vi "GSM调试.vi"() -> ()   [LabVIEW 2015]
doc: "GSM调试"
uses:
  <vilib>/Platform/browser.llb/Open URL in Default Browser (string).vi
  lib/pcomm/PCOMM.lvlib
panel:
  out "字符串 4":string="通用指令"
  out "字符串 3":string="串口设置"
  in  "刷新按钮":bool
  out "字符串 2":string="串口设置"
  in  "发送":string
  in  "打开/关闭串口":bool
  in  "波特率":i32(ring)=16 items=["1800"=8, "2400"=9, "4800"=10, "7200"=11, "9600"=12, "19200"=13, "38400"=14, "57600"=15, "115200"=16, "230400"=17, "460800"=18, "921600"=19]
  in  "数据比特":i32(ring)=3 caption="数据位" items=["5", "6", "7", "8"]
  in  "停止位":i32(ring) items=["1"=0, "2"=4]
  in  "奇偶校验":i32(ring) caption="校   验" items=["None"=0, "Odd"=8, "Even"=24, "Mark"=40, "Space"=56]
  in  "串口号":i32(ring)=1 items=["COM1 通信端口 (COM1)"=1, "COM2 ELTIMA Virtual Serial Port (COM2->COM5)"=2, "COM4 USB-SERIAL CH340 (COM4)"=4, "COM5 ELTIMA Virtual Serial Port (COM5->COM2)"=5]
  in  "打开文档":bool
  in  "清屏":bool
  in  "编号":u16
  in  "短信":string
  in  "号码":u64
  in  "显示回车换行":bool
  in  "GSM指令":T1={"响应测试"=FALSE, "版本信息"=FALSE, "查询IMEI"=FALSE, "信号质量查询"=FALSE, "本机号码"=FALSE, "显示ID"=FALSE, "呼叫号码"=FALSE, "查询短信状态"=FALSE, "查询温度"=FALSE, "查询音量"=FALSE, "默认配置"=FALSE, "查询运营商"=FALSE, "当前配置"=FALSE, "查询型号"=FALSE, "接听电话"=FALSE, "挂断电话"=FALSE, "读取短信"=FALSE, "删除短信"=FALSE, "删除全部短信"=FALSE, "发送短信"=FALSE, "信息显示"="", "字符串 4"="通用指令", "字符串 5"="通用指令"}
  out "接收文本框:":string
  out "TX:":i32 max=65535
  out "RX:":i32 max=1000
  in  "发送":bool
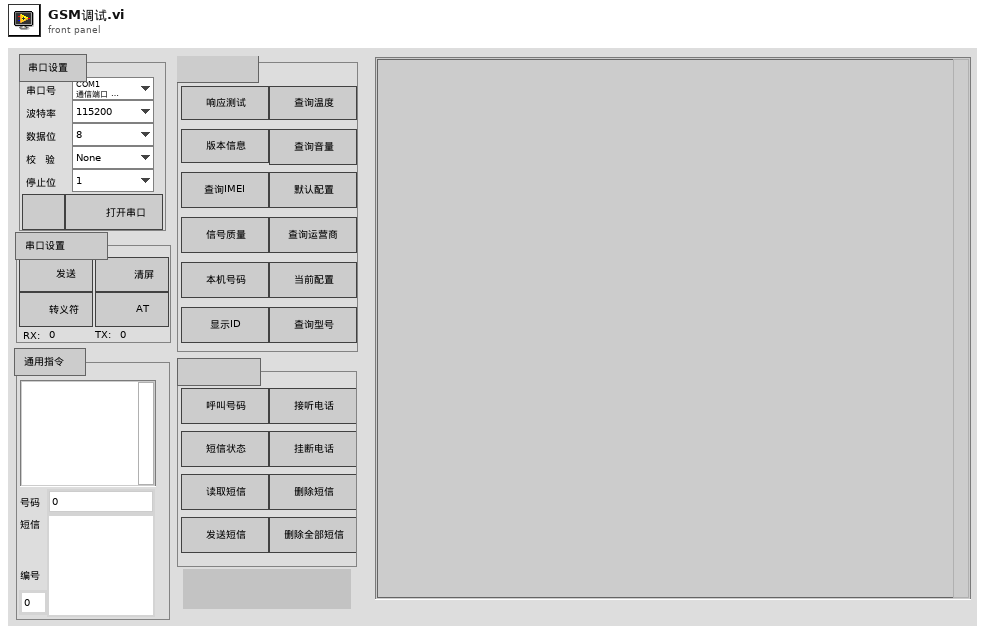
[diagram p1: front panel]
types:
  T1 = cluster{"响应测试":bool, "版本信息":bool, "查询IMEI":bool, "信号质量查询":bool, "本机号码":bool, "显示ID":bool, "呼叫号码":bool, "查询短信状态":bool, "查询温度":bool, "查询音量":bool, "默认配置":bool, "查询运营商":bool, "当前配置":bool, "查询型号":bool, "接听电话":bool, "挂断电话":bool, "读取短信":bool, "删除短信":bool, "删除全部短信":bool, "发送短信":bool, "信息显示":string, "字符串 4":string, "字符串 5":string}
  T2 = enum8{"Enabled", "Disabled", "Disabled and Grayed Out"}
  T3 = typedef "LVRectTypeDef.ctl" = cluster{"Left":i16, "Top":i16, "Right":i16, "Bottom":i16}
  T4 = typedef "LVPointTypeDef.ctl" = cluster{"Horizontal":i16, "Vertical":i16}
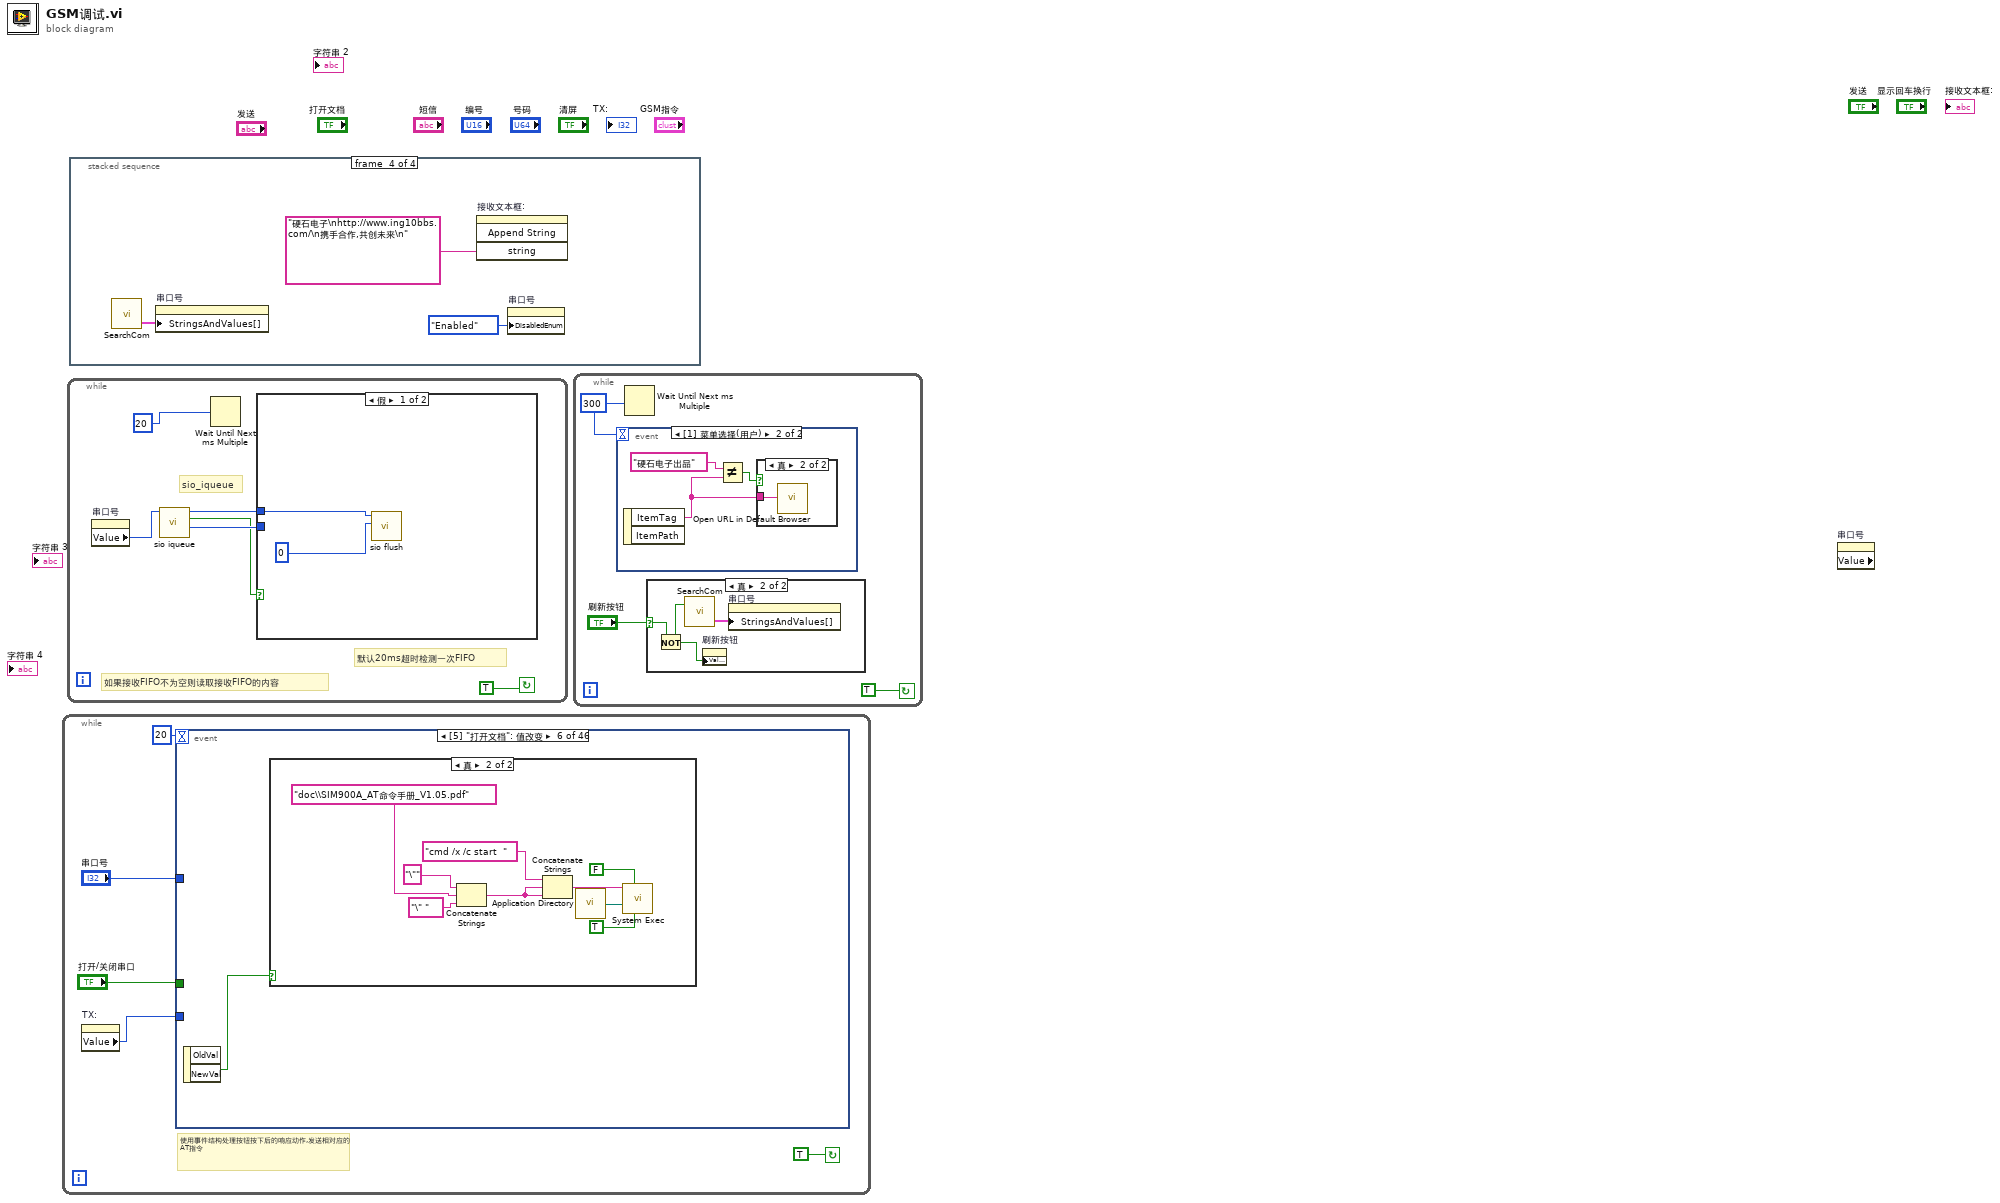
[diagram p0: block diagram]
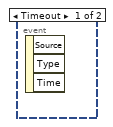
[diagram p3: hidden frame]
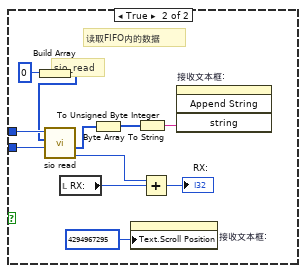
[diagram p5: hidden frame]
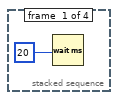
[diagram p6: hidden frame]
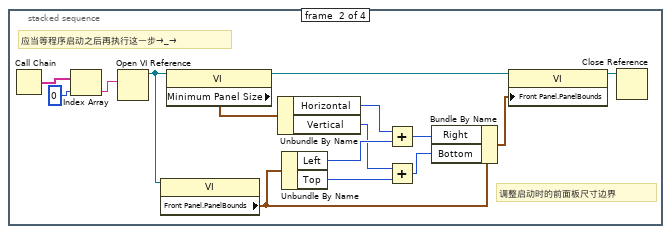
[diagram p7: hidden frame]
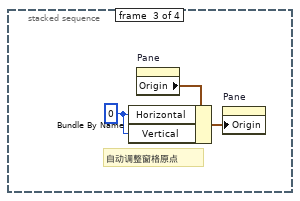
[diagram p8: hidden frame]
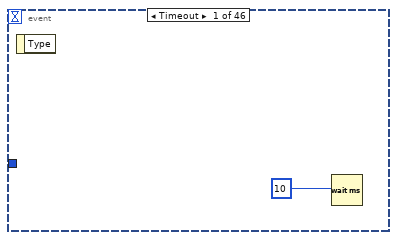
[diagram p9: hidden frame]
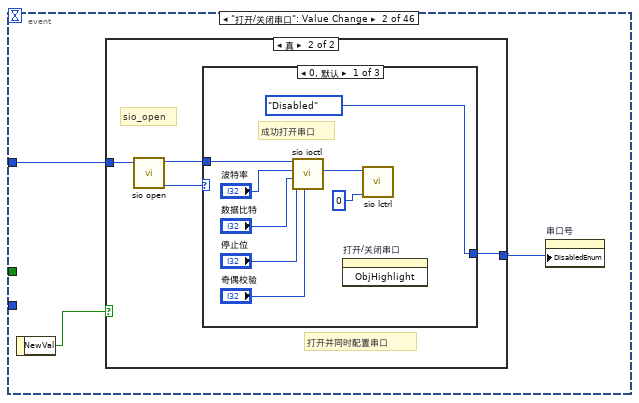
[diagram p10: hidden frame]
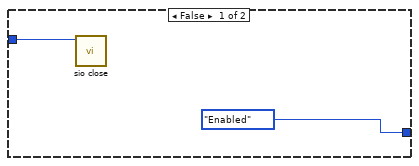
[diagram p11: hidden frame]
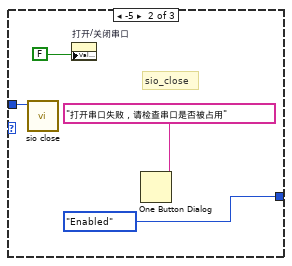
[diagram p12: hidden frame]
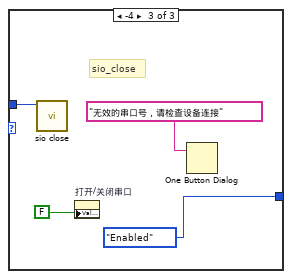
[diagram p13: hidden frame]
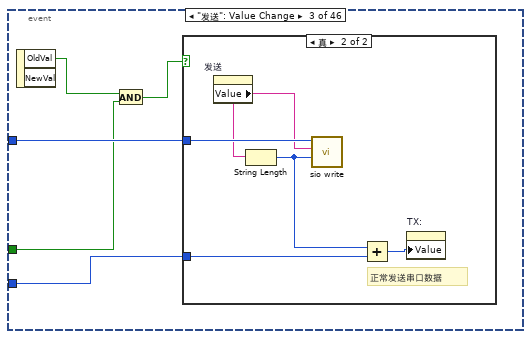
[diagram p14: hidden frame]
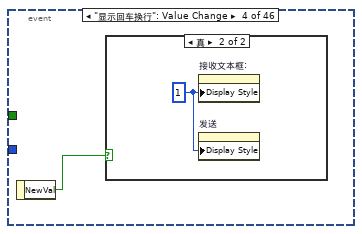
[diagram p16: hidden frame]
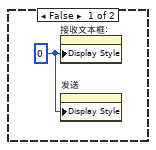
[diagram p17: hidden frame]
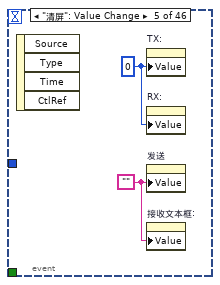
[diagram p18: hidden frame]
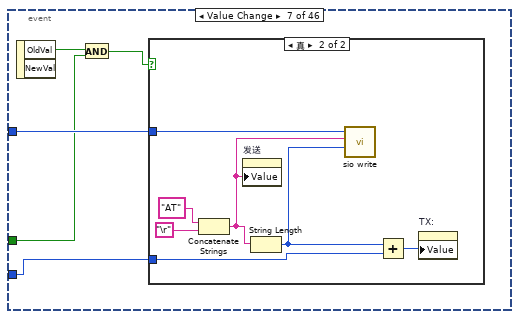
[diagram p20: hidden frame]
diagram:
  n1 = while {
    stop <- TRUE continue-if-true
    # "使用事件结构处理按钮按下后的响应动作,发送相对应的AT指令"
    n2 = property on="TX:" class="DigNum (严格)"() -> ("Value"=w4:i32)  [unwired: 2 in, 2 out]
    n3 = event shown="[5] \"打开文档\": 值改变" {
      selector: _ -> [_ _ _ _ _ _ _ _ _ _ _ _ _ _ _ _ _ _ _ _ _ _ _ _ _ _ _ _ _ _ _ _ _ _ _ _ _ _ _ _ _ _ _ _ _ _]
      dyn-events: _ -> [_ _ _ _ _ _ _ _ _ _ _ _ _ _ _ _ _ _ _ _ _ _ _ _ _ _ _ _ _ _ _ _ _ _ _ _ _ _ _ _ _ _ _ _ _ _]
      timeout: 20 -> [_ _ _ _ _ _ _ _ _ _ _ _ _ _ _ _ _ _ _ _ _ _ _ _ _ _ _ _ _ _ _ _ _ _ _ _ _ _ _ _ _ _ _ _ _ _]
      tunnel: w4 -> [_ _ w36 _ _ _ w61 w73 w85 w97 w109 w121 w133 w148 w160 w172 w184 w196 w208 w220 w232 w244 w256 w270 w284 w295 _ _ _ _ _ _ _ _ _ _ _ _ _ _ _ _ _ _ _ _]
      tunnel: "串口号" -> [_ w8 w35 _ _ _ w60 w72 w84 w96 w108 w120 w132 w147 w159 w171 w183 w195 w207 w219 w231 w243 w255 w269 w283 w296 _ _ _ _ _ _ _ _ _ _ _ _ _ _ _ _ _ _ _ _]
      tunnel: "打开/关闭串口" -> [_ _ w33 _ _ _ w58 w70 w82 w94 w106 w118 w130 w145 w157 w169 w181 w193 w205 w217 w229 w241 w253 w267 w281 w293 _ _ _ _ _ _ _ _ _ _ _ _ _ _ _ _ _ _ _ _]
      event Timeout {
        n4 = event-data() -> ()  [unwired: 1 in, 1 out]
        n5 = Wait (ms)(milliseconds to wait=10) -> ()  [unwired: 1 out]
      }
      event "打开/关闭串口": Value Change {
        n6 = event-data() -> ("NewVal"=w9:bool)  [unwired: 1 in]
        n7 = case shown="真" w9 {
          tunnel: w8 -> [w10 w12]
          tunnel: [T2."Enabled" w13] -> w7
          frame False {
            n8 = call "sio close.vi"("port"=w10) -> ()  [unwired: 9 in, 2 out]
          }
          frame True {
            # "sio_open"
            # "打开并同时配置串口"
            n9 = call "sio open.vi"("port"=w12) -> ("port"=w14:i32, "Status"=w15:i32)  [unwired: 6 in]
            n10 = case shown="0, 默认" w15 {
              tunnel: w14 -> [w19 w24 w28]
              tunnel: [T2."Disabled" T2."Enabled" T2."Enabled"] -> w13
              frame 0, Default {
                # "成功打开串口"
                n11 = call "sio ioctl.vi"("parity"="奇偶校验", "stop bits"="停止位", "data bits"="数据比特", "baud"="波特率", "port"=w19) -> ("port"=w17:i32)  [unwired: 5 in, 1 out]
                n12 = invoke on="打开/关闭串口" class="Bool (严格)" method="ObjHighlight"() -> ()  [unwired: 3 in, 3 out]
                n13 = call "sio lctrl.vi"("mode"=0, "port"=w17) -> ()  [unwired: 8 in, 2 out]
              }
              frame -5 {
                # "sio_close"
                n14 = call "sio close.vi"("port"=w24) -> ()  [unwired: 9 in, 2 out]
                n15 = property on="打开/关闭串口" class="Bool (严格)"("Value"=FALSE) -> ()  [unwired: 2 in, 2 out]
                n16 = One Button Dialog(message="打开串口失败，请检查串口是否被占用") -> ()  [unwired: 1 in, 1 out]
              }
              frame -4 {
                # "sio_close"
                n17 = call "sio close.vi"("port"=w28) -> ()  [unwired: 9 in, 2 out]
                n18 = property on="打开/关闭串口" class="Bool (严格)"("Value"=FALSE) -> ()  [unwired: 2 in, 2 out]
                n19 = One Button Dialog(message="无效的串口号，请检查设备连接") -> ()  [unwired: 1 in, 1 out]
              }
            }
          }
        }
        n20 = property on="串口号" class="Ring (严格)"("DisabledEnum"=w7) -> ()  [unwired: 2 in, 2 out]
      }
      event "发送": Value Change {
        n21 = event-data() -> ("OldVal"=w34:bool)  [unwired: 1 in, 1 out]
        n22 = And(x=w34, y=w33) -> (x .and. y?=w32:bool)
        n23 = case shown="真" w32 {
          tunnel: w35 -> [_ w39]
          tunnel: w36 -> [_ w41]
          frame False {
          }
          frame True {
            # "正常发送串口数据"
            n24 = property on="发送" class="Str"() -> ("Value"=w38:string)  [unwired: 2 in, 2 out]
            n25 = String Length(string=w38) -> (length=w37:i32)
            n26 = call "sio write.vi"("len"=w37, "buf"=w38, "port"=w39) -> ()  [unwired: 6 in, 3 out]
            n27 = Add(x=w37, y=w41) -> (x+y=w40:i32)
            n28 = property on="TX:" class="DigNum (严格)"("Value"=w40) -> ()  [unwired: 2 in, 2 out]
          }
        }
      }
      event "显示回车换行": Value Change {
        n29 = event-data() -> ("NewVal"=w42:bool)  [unwired: 1 in]
        n30 = case shown="真" w42 {
          frame False {
            w43 = u32 0
            n31 = property on="接收文本框:" class="Str"("Display Style"=w43) -> ()  [unwired: 2 in, 2 out]
            n32 = property on="发送" class="Str"("Display Style"=w43) -> ()  [unwired: 2 in, 2 out]
          }
          frame True {
            w44 = u32 1
            n33 = property on="接收文本框:" class="Str"("Display Style"=w44) -> ()  [unwired: 2 in, 2 out]
            n34 = property on="发送" class="Str"("Display Style"=w44) -> ()  [unwired: 2 in, 2 out]
          }
        }
      }
      event "清屏": Value Change {
        w45 = ""
        w46 = 0
        n35 = event-data() -> ()  [unwired: 1 in, 4 out]
        n36 = property on="TX:" class="DigNum (严格)"("Value"=w46) -> ()  [unwired: 2 in, 2 out]
        n37 = property on="RX:" class="DigNum (严格)"("Value"=w46) -> ()  [unwired: 2 in, 2 out]
        n38 = property on="发送" class="Str"("Value"=w45) -> ()  [unwired: 2 in, 2 out]
        n39 = property on="接收文本框:" class="Str"("Value"=w45) -> ()  [unwired: 2 in, 2 out]
      }
      event "打开文档": Value Change {
        n40 = event-data() -> ("NewVal"=w47:bool)  [unwired: 1 in, 1 out]
        n41 = case shown="真" w47 {
          frame False {
          }
          frame True {
            n42 = Concatenate Strings("\"" ("Substring"), "doc\\SIM900A_AT命令手册_V1.05.pdf", "\" " ("Substring")) -> (w53:string)
            n43 = Concatenate Strings("cmd /x /c start  ", w53, w53) -> (w55:string)
            n44 = call <vilib>:"Application Directory.vi"() -> ("Application Directory"=w48:path)
            n45 = call <vilib>:"System Exec.vi"("run minimized? (F)"=TRUE, "wait until completion? (T)"=FALSE ("Wait until done"), "working directory"=w48, "command line"=w55) -> ()  [unwired: 2 in, 6 out]
          }
        }
      }
      event "GSM指令.响应测试": Value Change {
        n46 = event-data() -> ("OldVal"=w59:bool)  [unwired: 1 in, 1 out]
        n47 = And(x=w59, y=w58) -> (x .and. y?=w57:bool)
        n48 = case shown="真" w57 {
          tunnel: w60 -> [_ w64]
          tunnel: w61 -> [_ w67]
          frame False {
          }
          frame True {
            n49 = Concatenate Strings("AT", "\r") -> (w63:string)
            n50 = property on="发送" class="Str"("Value"=w63) -> ()  [unwired: 2 in, 2 out]
            n51 = String Length(string=w63) -> (length=w62:i32)
            n52 = call "sio write.vi"("len"=w62, "buf"=w63, "port"=w64) -> ()  [unwired: 6 in, 3 out]
            n53 = Add(x=w62, y=w67) -> (x+y=w68:i32)
            n54 = property on="TX:" class="DigNum (严格)"("Value"=w68) -> ()  [unwired: 2 in, 2 out]
          }
        }
      }
      event "GSM指令.版本信息": Value Change {
        n55 = event-data() -> ("OldVal"=w69:bool)  [unwired: 1 in, 1 out]
        n56 = And(x=w70, y=w69) -> (x .and. y?=w71:bool)
        n57 = case shown="真" w71 {
          tunnel: w72 -> [_ w76]
          tunnel: w73 -> [_ w79]
          frame False {
          }
          frame True {
            n58 = Concatenate Strings("AT+GSV", "\r") -> (w75:string)
            n59 = property on="发送" class="Str"("Value"=w75) -> ()  [unwired: 2 in, 2 out]
            n60 = String Length(string=w75) -> (length=w74:i32)
            n61 = call "sio write.vi"("len"=w74, "buf"=w75, "port"=w76) -> ()  [unwired: 6 in, 3 out]
            n62 = Add(x=w74, y=w79) -> (x+y=w80:i32)
            n63 = property on="TX:" class="DigNum (严格)"("Value"=w80) -> ()  [unwired: 2 in, 2 out]
          }
        }
      }
      event "GSM指令.查询IMEI": Value Change {
        n64 = event-data() -> ("OldVal"=w83:bool)  [unwired: 1 in, 1 out]
        n65 = And(x=w83, y=w82) -> (x .and. y?=w81:bool)
        n66 = case shown="真" w81 {
          tunnel: w84 -> [_ w88]
          tunnel: w85 -> [_ w91]
          frame False {
          }
          frame True {
            n67 = Concatenate Strings("AT+GSN", "\r") -> (w87:string)
            n68 = property on="发送" class="Str"("Value"=w87) -> ()  [unwired: 2 in, 2 out]
            n69 = String Length(string=w87) -> (length=w86:i32)
            n70 = call "sio write.vi"("len"=w86, "buf"=w87, "port"=w88) -> ()  [unwired: 6 in, 3 out]
            n71 = Add(x=w86, y=w91) -> (x+y=w92:i32)
            n72 = property on="TX:" class="DigNum (严格)"("Value"=w92) -> ()  [unwired: 2 in, 2 out]
          }
        }
      }
      event "GSM指令.信号质量查询": Value Change {
        n73 = event-data() -> ("OldVal"=w95:bool)  [unwired: 1 in, 1 out]
        n74 = And(x=w95, y=w94) -> (x .and. y?=w93:bool)
        n75 = case shown="真" w93 {
          tunnel: w96 -> [_ w100]
          tunnel: w97 -> [_ w103]
          frame False {
          }
          frame True {
            n76 = Concatenate Strings("AT+CSQ", "\r") -> (w99:string)
            n77 = property on="发送" class="Str"("Value"=w99) -> ()  [unwired: 2 in, 2 out]
            n78 = String Length(string=w99) -> (length=w98:i32)
            n79 = call "sio write.vi"("len"=w98, "buf"=w99, "port"=w100) -> ()  [unwired: 6 in, 3 out]
            n80 = Add(x=w98, y=w103) -> (x+y=w104:i32)
            n81 = property on="TX:" class="DigNum (严格)"("Value"=w104) -> ()  [unwired: 2 in, 2 out]
          }
        }
      }
      event "GSM指令.本机号码": Value Change {
        n82 = event-data() -> ("OldVal"=w107:bool)  [unwired: 1 in, 1 out]
        n83 = And(x=w107, y=w106) -> (x .and. y?=w105:bool)
        n84 = case shown="真" w105 {
          tunnel: w108 -> [_ w112]
          tunnel: w109 -> [_ w115]
          frame False {
          }
          frame True {
            n85 = Concatenate Strings("AT+CNUM", "\r") -> (w111:string)
            n86 = String Length(string=w111) -> (length=w110:i32)
            n87 = property on="发送" class="Str"("Value"=w111) -> ()  [unwired: 2 in, 2 out]
            n88 = call "sio write.vi"("len"=w110, "buf"=w111, "port"=w112) -> ()  [unwired: 6 in, 3 out]
            n89 = Add(x=w110, y=w115) -> (x+y=w116:i32)
            n90 = property on="TX:" class="DigNum (严格)"("Value"=w116) -> ()  [unwired: 2 in, 2 out]
          }
        }
      }
      event "GSM指令.显示ID": Value Change {
        n91 = event-data() -> ("OldVal"=w119:bool)  [unwired: 1 in, 1 out]
        n92 = And(x=w119, y=w118) -> (x .and. y?=w117:bool)
        n93 = case shown="真" w117 {
          tunnel: w120 -> [_ w124]
          tunnel: w121 -> [_ w127]
          frame False {
          }
          frame True {
            n94 = Concatenate Strings("ATI", "\r") -> (w123:string)
            n95 = property on="发送" class="Str"("Value"=w123) -> ()  [unwired: 2 in, 2 out]
            n96 = String Length(string=w123) -> (length=w122:i32)
            n97 = call "sio write.vi"("len"=w122, "buf"=w123, "port"=w124) -> ()  [unwired: 6 in, 3 out]
            n98 = Add(x=w122, y=w127) -> (x+y=w128:i32)
            n99 = property on="TX:" class="DigNum (严格)"("Value"=w128) -> ()  [unwired: 2 in, 2 out]
          }
        }
      }
      event "GSM指令.呼叫号码": Value Change {
        n100 = event-data() -> ("OldVal"=w131:bool)  [unwired: 1 in, 1 out]
        n101 = And(x=w131, y=w130) -> (x .and. y?=w129:bool)
        n102 = case shown="真" w129 {
          tunnel: w132 -> [_ w136]
          tunnel: w133 -> [_ w142]
          frame False {
          }
          frame True {
            n103 = property on="号码" class="DigNum (严格)"() -> ("Value"=w138:u64)  [unwired: 2 in, 2 out]
            n104 = Number To Decimal String ("数值至十进制数字符串转换")(number=w138) -> (decimal integer string=w140:string)  [unwired: 1 in]
            n105 = Concatenate Strings("ATD", w140, ";", "\r") -> (w135:string)
            n106 = property on="发送" class="Str"("Value"=w135) -> ()  [unwired: 2 in, 2 out]
            n107 = String Length(string=w135) -> (length=w134:i32)
            n108 = call "sio write.vi"("len"=w134, "buf"=w135, "port"=w136) -> ()  [unwired: 6 in, 3 out]
            n109 = Add(x=w134, y=w142) -> (x+y=w143:i32)
            n110 = property on="TX:" class="DigNum (严格)"("Value"=w143) -> ()  [unwired: 2 in, 2 out]
          }
        }
      }
      event "GSM指令.查询短信状态": Value Change {
        n111 = event-data() -> ("OldVal"=w146:bool)  [unwired: 1 in, 1 out]
        n112 = And(x=w146, y=w145) -> (x .and. y?=w144:bool)
        n113 = case shown="真" w144 {
          tunnel: w147 -> [_ w151]
          tunnel: w148 -> [_ w154]
          frame False {
          }
          frame True {
            n114 = Concatenate Strings("AT+CPMS?", "\r") -> (w150:string)
            n115 = property on="发送" class="Str"("Value"=w150) -> ()  [unwired: 2 in, 2 out]
            n116 = String Length(string=w150) -> (length=w149:i32)
            n117 = Add(x=w149, y=w154) -> (x+y=w155:i32)
            n118 = call "sio write.vi"("len"=w149, "buf"=w150, "port"=w151) -> ()  [unwired: 6 in, 3 out]
            n119 = property on="TX:" class="DigNum (严格)"("Value"=w155) -> ()  [unwired: 2 in, 2 out]
          }
        }
      }
      event "GSM指令.查询温度": Value Change {
        n120 = event-data() -> ("OldVal"=w158:bool)  [unwired: 1 in, 1 out]
        n121 = And(x=w158, y=w157) -> (x .and. y?=w156:bool)
        n122 = case shown="真" w156 {
          tunnel: w159 -> [_ w163]
          tunnel: w160 -> [_ w166]
          frame False {
          }
          frame True {
            n123 = Concatenate Strings("AT+CMTE?", "\r") -> (w162:string)
            n124 = property on="发送" class="Str"("Value"=w162) -> ()  [unwired: 2 in, 2 out]
            n125 = String Length(string=w162) -> (length=w161:i32)
            n126 = Add(x=w161, y=w166) -> (x+y=w167:i32)
            n127 = call "sio write.vi"("len"=w161, "buf"=w162, "port"=w163) -> ()  [unwired: 6 in, 3 out]
            n128 = property on="TX:" class="DigNum (严格)"("Value"=w167) -> ()  [unwired: 2 in, 2 out]
          }
        }
      }
      event "GSM指令.查询音量": Value Change {
        n129 = event-data() -> ("OldVal"=w170:bool)  [unwired: 1 in, 1 out]
        n130 = And(x=w170, y=w169) -> (x .and. y?=w168:bool)
        n131 = case shown="真" w168 {
          tunnel: w171 -> [_ w175]
          tunnel: w172 -> [_ w178]
          frame False {
          }
          frame True {
            n132 = Concatenate Strings("AT+SIDET?", "\r") -> (w174:string)
            n133 = property on="发送" class="Str"("Value"=w174) -> ()  [unwired: 2 in, 2 out]
            n134 = String Length(string=w174) -> (length=w173:i32)
            n135 = call "sio write.vi"("len"=w173, "buf"=w174, "port"=w175) -> ()  [unwired: 6 in, 3 out]
            n136 = Add(x=w173, y=w178) -> (x+y=w179:i32)
            n137 = property on="TX:" class="DigNum (严格)"("Value"=w179) -> ()  [unwired: 2 in, 2 out]
          }
        }
      }
      event "GSM指令.默认配置": Value Change {
        n138 = event-data() -> ("OldVal"=w182:bool)  [unwired: 1 in, 1 out]
        n139 = And(x=w182, y=w181) -> (x .and. y?=w180:bool)
        n140 = case shown="真" w180 {
          tunnel: w183 -> [_ w187]
          tunnel: w184 -> [_ w190]
          frame False {
          }
          frame True {
            n141 = Concatenate Strings("AT&F", "\r") -> (w186:string)
            n142 = property on="发送" class="Str"("Value"=w186) -> ()  [unwired: 2 in, 2 out]
            n143 = String Length(string=w186) -> (length=w185:i32)
            n144 = call "sio write.vi"("len"=w185, "buf"=w186, "port"=w187) -> ()  [unwired: 6 in, 3 out]
            n145 = Add(x=w185, y=w190) -> (x+y=w191:i32)
            n146 = property on="TX:" class="DigNum (严格)"("Value"=w191) -> ()  [unwired: 2 in, 2 out]
          }
        }
      }
      event "GSM指令.查询运营商": Value Change {
        n147 = event-data() -> ("OldVal"=w194:bool)  [unwired: 1 in, 1 out]
        n148 = And(x=w194, y=w193) -> (x .and. y?=w192:bool)
        n149 = case shown="真" w192 {
          tunnel: w195 -> [_ w199]
          tunnel: w196 -> [_ w202]
          frame False {
          }
          frame True {
            n150 = Concatenate Strings("AT+COPS?", "\r") -> (w198:string)
            n151 = property on="发送" class="Str"("Value"=w198) -> ()  [unwired: 2 in, 2 out]
            n152 = String Length(string=w198) -> (length=w197:i32)
            n153 = call "sio write.vi"("len"=w197, "buf"=w198, "port"=w199) -> ()  [unwired: 6 in, 3 out]
            n154 = Add(x=w197, y=w202) -> (x+y=w203:i32)
            n155 = property on="TX:" class="DigNum (严格)"("Value"=w203) -> ()  [unwired: 2 in, 2 out]
          }
        }
      }
      event "GSM指令.当前配置": Value Change {
        n156 = event-data() -> ("OldVal"=w206:bool)  [unwired: 1 in, 1 out]
        n157 = And(x=w206, y=w205) -> (x .and. y?=w204:bool)
        n158 = case shown="真" w204 {
          tunnel: w207 -> [_ w211]
          tunnel: w208 -> [_ w214]
          frame False {
          }
          frame True {
            n159 = Concatenate Strings("AT&V", "\r") -> (w210:string)
            n160 = property on="发送" class="Str"("Value"=w210) -> ()  [unwired: 2 in, 2 out]
            n161 = String Length(string=w210) -> (length=w209:i32)
            n162 = call "sio write.vi"("len"=w209, "buf"=w210, "port"=w211) -> ()  [unwired: 6 in, 3 out]
            n163 = Add(x=w209, y=w214) -> (x+y=w215:i32)
            n164 = property on="TX:" class="DigNum (严格)"("Value"=w215) -> ()  [unwired: 2 in, 2 out]
          }
        }
      }
      event "GSM指令.查询型号": Value Change {
        n165 = event-data() -> ("OldVal"=w218:bool)  [unwired: 1 in, 1 out]
        n166 = And(x=w218, y=w217) -> (x .and. y?=w216:bool)
        n167 = case shown="真" w216 {
          tunnel: w219 -> [_ w223]
          tunnel: w220 -> [_ w226]
          frame False {
          }
          frame True {
            n168 = Concatenate Strings("AT+CGMM", "\r") -> (w222:string)
            n169 = property on="发送" class="Str"("Value"=w222) -> ()  [unwired: 2 in, 2 out]
            n170 = String Length(string=w222) -> (length=w221:i32)
            n171 = call "sio write.vi"("len"=w221, "buf"=w222, "port"=w223) -> ()  [unwired: 6 in, 3 out]
            n172 = Add(x=w221, y=w226) -> (x+y=w227:i32)
            n173 = property on="TX:" class="DigNum (严格)"("Value"=w227) -> ()  [unwired: 2 in, 2 out]
          }
        }
      }
      event "GSM指令.接听电话": Value Change {
        n174 = event-data() -> ("OldVal"=w230:bool)  [unwired: 1 in, 1 out]
        n175 = And(x=w230, y=w229) -> (x .and. y?=w228:bool)
        n176 = case shown="真" w228 {
          tunnel: w232 -> [_ w238]
          tunnel: w231 -> [_ w235]
          frame False {
          }
          frame True {
            n177 = Concatenate Strings("ATA", "\r") -> (w234:string)
            n178 = property on="发送" class="Str"("Value"=w234) -> ()  [unwired: 2 in, 2 out]
            n179 = String Length(string=w234) -> (length=w233:i32)
            n180 = call "sio write.vi"("len"=w233, "buf"=w234, "port"=w235) -> ()  [unwired: 6 in, 3 out]
            n181 = Add(x=w233, y=w238) -> (x+y=w239:i32)
            n182 = property on="TX:" class="DigNum (严格)"("Value"=w239) -> ()  [unwired: 2 in, 2 out]
          }
        }
      }
      event "GSM指令.挂断电话": Value Change {
        n183 = event-data() -> ("OldVal"=w242:bool)  [unwired: 1 in, 1 out]
        n184 = And(x=w242, y=w241) -> (x .and. y?=w240:bool)
        n185 = case shown="真" w240 {
          tunnel: w244 -> [_ w250]
          tunnel: w243 -> [_ w247]
          frame False {
          }
          frame True {
            n186 = Concatenate Strings("ATH", "\r") -> (w246:string)
            n187 = property on="发送" class="Str"("Value"=w246) -> ()  [unwired: 2 in, 2 out]
            n188 = String Length(string=w246) -> (length=w245:i32)
            n189 = call "sio write.vi"("len"=w245, "buf"=w246, "port"=w247) -> ()  [unwired: 6 in, 3 out]
            n190 = Add(x=w245, y=w250) -> (x+y=w251:i32)
            n191 = property on="TX:" class="DigNum (严格)"("Value"=w251) -> ()  [unwired: 2 in, 2 out]
          }
        }
      }
      event "GSM指令.读取短信": Value Change {
        n192 = event-data() -> ("OldVal"=w254:bool)  [unwired: 1 in, 1 out]
        n193 = And(x=w254, y=w253) -> (x .and. y?=w252:bool)
        n194 = case shown="真" w252 {
          tunnel: w256 -> [_ w264]
          tunnel: w255 -> [_ w259]
          frame False {
          }
          frame True {
            n195 = property on="编号" class="DigNum (严格)"() -> ("Value"=w261:u16)  [unwired: 2 in, 2 out]
            n196 = Number To Decimal String(number=w261) -> (decimal integer string=w262:string)  [unwired: 1 in]
            n197 = Concatenate Strings("AT+CMGR=", w262, "\r") -> (w258:string)
            n198 = property on="发送" class="Str"("Value"=w258) -> ()  [unwired: 2 in, 2 out]
            n199 = String Length(string=w258) -> (length=w257:i32)
            n200 = Add(x=w257, y=w264) -> (x+y=w265:i32)
            n201 = call "sio write.vi"("len"=w257, "buf"=w258, "port"=w259) -> ()  [unwired: 6 in, 3 out]
            n202 = property on="TX:" class="DigNum (严格)"("Value"=w265) -> ()  [unwired: 2 in, 2 out]
          }
        }
      }
      event "GSM指令.删除短信": Value Change {
        n203 = event-data() -> ("OldVal"=w268:bool)  [unwired: 1 in, 1 out]
        n204 = And(x=w268, y=w267) -> (x .and. y?=w266:bool)
        n205 = case shown="真" w266 {
          tunnel: w270 -> [_ w278]
          tunnel: w269 -> [_ w273]
          frame False {
          }
          frame True {
            n206 = property on="编号" class="DigNum (严格)"() -> ("Value"=w275:u16)  [unwired: 2 in, 2 out]
            n207 = Number To Decimal String(number=w275) -> (decimal integer string=w276:string)  [unwired: 1 in]
            n208 = Concatenate Strings("AT+CMGD=", w276, "\r") -> (w272:string)
            n209 = property on="发送" class="Str"("Value"=w272) -> ()  [unwired: 2 in, 2 out]
            n210 = String Length(string=w272) -> (length=w271:i32)
            n211 = call "sio write.vi"("len"=w271, "buf"=w272, "port"=w273) -> ()  [unwired: 6 in, 3 out]
            n212 = Add(x=w271, y=w278) -> (x+y=w279:i32)
            n213 = property on="TX:" class="DigNum (严格)"("Value"=w279) -> ()  [unwired: 2 in, 2 out]
          }
        }
      }
      event "GSM指令.删除全部短信": Value Change {
        n214 = event-data() -> ("OldVal"=w282:bool)  [unwired: 1 in, 1 out]
        n215 = And(x=w282, y=w281) -> (x .and. y?=w280:bool)
        n216 = case shown="真" w280 {
          tunnel: w284 -> [_ w290]
          tunnel: w283 -> [_ w287]
          frame False {
          }
          frame True {
            n217 = Concatenate Strings("AT+CMGDA=\"DEL ALL\"", "\r") -> (w286:string)
            n218 = property on="发送" class="Str"("Value"=w286) -> ()  [unwired: 2 in, 2 out]
            n219 = String Length(string=w286) -> (length=w285:i32)
            n220 = call "sio write.vi"("len"=w285, "buf"=w286, "port"=w287) -> ()  [unwired: 6 in, 3 out]
            n221 = Add(x=w285, y=w290) -> (x+y=w291:i32)
            n222 = property on="TX:" class="DigNum (严格)"("Value"=w291) -> ()  [unwired: 2 in, 2 out]
          }
        }
      }
      event "GSM指令.发送短信": Value Change {
        # "短信以0x1A结束,\n就是十进制26"
        n223 = event-data() -> ("OldVal"=w294:bool)  [unwired: 1 in, 1 out]
        n224 = And(x=w294, y=w293) -> (x .and. y?=w292:bool)
        n225 = case shown="真" w292 {
          tunnel: w296 -> [_ w304]
          tunnel: w295 -> [_ w303]
          frame False {
          }
          frame True {
            n226 = stacked-sequence {
              tunnel: w304 -> [w307 _ w314 _ w321 _ w328 _ w338]
              tunnel: w303 -> [w308 _ w315 _ w322 _ w334 _ w343]
              tunnel: [_ _ _ _ _ _ w327 _ _] -> w298
              tunnel: [_ _ _ _ _ _ _ _ w337] -> w297
              tunnel: [_ _ w313 _ _ _ _ _ _] -> w300
              tunnel: [w306 _ _ _ _ _ _ _ _] -> w301
              tunnel: [_ _ _ _ w320 _ _ _ _] -> w299
              frame #0 {
                # "设置GSM字符集"
                n227 = Concatenate Strings("AT+CSCS=\"GSM\"", "\r") -> (w306:string)
                n228 = String Length(string=w306) -> (length=w305:i32)
                n229 = call "sio write.vi"("len"=w305, "buf"=w306, "port"=w307) -> ()  [unwired: 6 in, 3 out]
                n230 = Add(x=w305, y=w308) -> (x+y=w311:i32)
                n231 = property on="TX:" class="DigNum (严格)"("Value"=w311) -> ()  [unwired: 2 in, 2 out]
              }
              frame #1 {
                # "发送电话号码之后\n需要等待回复才能\n发送短信内容,这里\n延时10ms"
                n232 = call "时间延迟2"() -> ()  [unwired: 11 in, 1 out]
              }
              frame #2 {
                # "设置为文本模式"
                n233 = Concatenate Strings("AT+CMGF=1", "\r") -> (w313:string)
                n234 = String Length(string=w313) -> (length=w312:i32)
                n235 = call "sio write.vi"("len"=w312, "buf"=w313, "port"=w314) -> ()  [unwired: 6 in, 3 out]
                n236 = Add(x=w312, y=w315) -> (x+y=w318:i32)
                n237 = property on="TX:" class="DigNum (严格)"("Value"=w318) -> ()  [unwired: 2 in, 2 out]
              }
              frame #3 {
                # "发送电话号码之后\n需要等待回复才能\n发送短信内容,这里\n延时10ms"
                n238 = call "时间延迟5"() -> ()  [unwired: 11 in, 1 out]
              }
              frame #4 {
                # "设置文本模式参数"
                n239 = Concatenate Strings("AT+CSMP=17,167,0,8", "\r") -> (w320:string)
                n240 = String Length(string=w320) -> (length=w319:i32)
                n241 = call "sio write.vi"("len"=w319, "buf"=w320, "port"=w321) -> ()  [unwired: 6 in, 3 out]
                n242 = Add(x=w319, y=w322) -> (x+y=w325:i32)
                n243 = property on="TX:" class="DigNum (严格)"("Value"=w325) -> ()  [unwired: 2 in, 2 out]
              }
              frame #5 {
                # "每条指令发送时候\n需要等待响应,这里\n延时10ms"
                n244 = call "时间延迟3"() -> ()  [unwired: 11 in, 1 out]
              }
              frame #6 {
                # "发送号码"
                n245 = property on="号码" class="DigNum (严格)"() -> ("Value"=w331:u64)  [unwired: 2 in, 2 out]
                n246 = Number To Decimal String ("数值至十进制数字符串转换")(number=w331) -> (decimal integer string=w332:string)  [unwired: 1 in]
                n247 = Concatenate Strings("AT+CMGS=\"", w332, "\"", "\r") -> (w327:string)
                n248 = String Length(string=w327) -> (length=w326:i32)
                n249 = call "sio write.vi"("len"=w326, "buf"=w327, "port"=w328) -> ()  [unwired: 6 in, 3 out]
                n250 = Add(x=w326, y=w334) -> (x+y=w335:i32)
                n251 = property on="TX:" class="DigNum (严格)"("Value"=w335) -> ()  [unwired: 2 in, 2 out]
              }
              frame #7 {
                # "发送电话号码之后\n需要等待回复才能\n发送短信内容,这里\n延时10ms"
                n252 = call "时间延迟"() -> ()  [unwired: 11 in, 1 out]
              }
              frame #8 {
                # "发送短信内容"
                n253 = property on="短信" class="Str"() -> ("Value"=w339:string)  [unwired: 2 in, 2 out]
                n254 = Type Cast(type=w339, x=u8 26) -> (*(type *) &x=w341:string)
                n255 = Concatenate Strings(w339, w341) -> (w337:string)
                n256 = String Length(string=w337) -> (length=w336:i32)
                n257 = call "sio write.vi"("len"=w336, "buf"=w337, "port"=w338) -> ()  [unwired: 6 in, 3 out]
                n258 = Add(x=w336, y=w343) -> (x+y=w342:i32)
                n259 = property on="TX:" class="DigNum (严格)"("Value"=w342) -> ()  [unwired: 2 in, 2 out]
              }
            }
            n260 = Concatenate Strings(w301, w300, w299, w298, w297) -> (w302:string)
            n261 = property on="发送" class="Str"("Value"=w302) -> ()  [unwired: 2 in, 2 out]
          }
        }
      }
      event "GSM指令.响应测试": Mouse Enter {
        n262 = event-data() -> ()  [unwired: 1 in, 1 out]
        n263 = property on="信息显示" class="Str"("Value"="测试模块是否正常连接") -> ()  [unwired: 2 in, 2 out]
      }
      event "GSM指令.版本信息": Mouse Enter {
        n264 = event-data() -> ()  [unwired: 1 in, 4 out]
        n265 = property on="信息显示" class="Str"("Value"="显示产品标识信息") -> ()  [unwired: 2 in, 2 out]
      }
      event "GSM指令.查询IMEI": Mouse Enter {
        n266 = event-data() -> ()  [unwired: 1 in, 4 out]
        n267 = property on="信息显示" class="Str"("Value"="查询TA序列号(IMEI)") -> ()  [unwired: 2 in, 2 out]
      }
      event "GSM指令.信号质量查询": Mouse Enter {
        n268 = event-data() -> ()  [unwired: 1 in, 4 out]
        n269 = property on="信息显示" class="Str"("Value"="信号质量查询") -> ()  [unwired: 2 in, 2 out]
      }
      event "GSM指令.本机号码": Mouse Enter {
        n270 = event-data() -> ()  [unwired: 1 in, 4 out]
        n271 = property on="信息显示" class="Str"("Value"="查询本机SIM卡号码") -> ()  [unwired: 2 in, 2 out]
      }
      event "GSM指令.显示ID": Mouse Enter {
        n272 = event-data() -> ()  [unwired: 1 in, 4 out]
        n273 = property on="信息显示" class="Str"("Value"="显示产品信息,例如:\nSIM900 11.0") -> ()  [unwired: 2 in, 2 out]
      }
      event "GSM指令.呼叫号码": Mouse Enter {
        n274 = event-data() -> ()  [unwired: 1 in, 4 out]
        n275 = property on="信息显示" class="Str"("Value"="发起一个语音呼叫") -> ()  [unwired: 2 in, 2 out]
      }
      event "GSM指令.查询短信状态": Mouse Enter {
        n276 = event-data() -> ()  [unwired: 1 in, 4 out]
        n277 = property on="信息显示" class="Str"("Value"="查询SIM卡消息存储器的状态\n响应:当前消息的数量,可存储的消息数量") -> ()  [unwired: 2 in, 2 out]
      }
      event "GSM指令.查询温度": Mouse Enter {
        n278 = event-data() -> ()  [unwired: 1 in, 4 out]
        n279 = property on="信息显示" class="Str"("Value"="查询模块温度") -> ()  [unwired: 2 in, 2 out]
      }
      event "GSM指令.查询音量": Mouse Enter {
        n280 = event-data() -> ()  [unwired: 1 in, 4 out]
        n281 = property on="信息显示" class="Str"("Value"="查询侧音增益等级\n响应:各通道的侧音增益等级") -> ()  [unwired: 2 in, 2 out]
      }
      event "GSM指令.默认配置": Mouse Enter {
        n282 = event-data() -> ()  [unwired: 1 in, 4 out]
        n283 = property on="信息显示" class="Str"("Value"="设置所有参数为出厂默认配置") -> ()  [unwired: 2 in, 2 out]
      }
      event "GSM指令.查询运营商": Mouse Enter {
        n284 = event-data() -> ()  [unwired: 1 in, 4 out]
        n285 = property on="信息显示" class="Str"("Value"="查询当前的模式和当前选择的运营商") -> ()  [unwired: 2 in, 2 out]
      }
      event "GSM指令.当前配置": Mouse Enter {
        n286 = event-data() -> ()  [unwired: 1 in, 4 out]
        n287 = property on="信息显示" class="Str"("Value"="显示当前配置") -> ()  [unwired: 2 in, 2 out]
      }
      event "GSM指令.查询型号": Mouse Enter {
        n288 = event-data() -> ()  [unwired: 1 in, 4 out]
        n289 = property on="信息显示" class="Str"("Value"="查询SIM模块型号") -> ()  [unwired: 2 in, 2 out]
      }
      event "GSM指令.接听电话": Mouse Enter {
        n290 = event-data() -> ()  [unwired: 1 in, 4 out]
        n291 = property on="信息显示" class="Str"("Value"="呼叫应答,当SIM模块主动上传:RING的时候才有效") -> ()  [unwired: 2 in, 2 out]
      }
      event "GSM指令.挂断电话": Mouse Enter {
        n292 = event-data() -> ()  [unwired: 1 in, 4 out]
        n293 = property on="信息显示" class="Str"("Value"="挂断当前呼叫连接") -> ()  [unwired: 2 in, 2 out]
      }
      event "GSM指令.读取短信": Mouse Enter {
        n294 = event-data() -> ()  [unwired: 1 in, 4 out]
        n295 = property on="信息显示" class="Str"("Value"="读取指定编号的短信") -> ()  [unwired: 2 in, 2 out]
      }
      event "GSM指令.删除短信": Mouse Enter {
        n296 = event-data() -> ()  [unwired: 1 in, 4 out]
        n297 = property on="信息显示" class="Str"("Value"="删除消息存储器中指定编号的短消息") -> ()  [unwired: 2 in, 2 out]
      }
      event "GSM指令.删除全部短信": Mouse Enter {
        n298 = event-data() -> ()  [unwired: 1 in, 4 out]
        n299 = property on="信息显示" class="Str"("Value"="删除所有短信") -> ()  [unwired: 2 in, 2 out]
      }
      event "GSM指令.发送短信": Mouse Enter {
        n300 = event-data() -> ()  [unwired: 1 in, 4 out]
        n301 = property on="信息显示" class="Str"("Value"="往指定号码发送短信\n暂时不支持中文短息发送") -> ()  [unwired: 2 in, 2 out]
      }
    }
  }
  n302 = while {
    stop <- TRUE continue-if-true
    # "sio_iqueue"
    # "如果接收FIFO不为空则读取接收FIFO的内容"
    # "默认20ms超时检测一次FIFO"
    n303 = property on="串口号" class="Ring (严格)"() -> ("Value"=w366:i32)  [unwired: 2 in, 2 out]
    n304 = call "sio iqueue.vi"("port"=w366) -> ("len"=w368:i32, "bool"=w364:bool, "port"=w365:i32)  [unwired: 8 in]
    n305 = Wait Until Next ms Multiple(millisecond multiple=u32 20) -> ()  [unwired: 1 out]
    n306 = case shown="假" w364 {
      tunnel: w365 -> [w370 w376]
      tunnel: w368 -> [_ w375]
      frame False {
        n307 = call "sio flush.vi"("func"=0, "port"=w370) -> ()  [unwired: 8 in, 2 out]
      }
      frame True {
        # "读取FIFO内的数据"
        # "sio_read"
        n308 = Build Array(i8 0) -> (w374:i8[])
        n309 = call "sio read.vi"("len"=w375, "buf"=w374, "port"=w376) -> ("len"=w372:i32, "buf out"=w373:i8[])  [unwired: 4 in, 2 out]
        n310 = local read "RX:"() -> (w381:i32)
        n311 = To Unsigned Byte Integer(number=w373) -> (unsigned 8bit integer=w378:u8[])
        n312 = property on="接收文本框:" class="Str"("Text.Scroll Position"=u32 4294967295) -> ()  [unwired: 2 in, 2 out]
        n313 = Byte Array To String(unsigned byte array=w378) -> (string=w377:string)
        n314 = Add(x=w372, y=w381) -> (x+y=→"RX:":i32)
        n315 = invoke on="接收文本框:" class="Str" method="Append String"("string"=w377) -> ()  [unwired: 3 in, 4 out]
      }
    }
  }
  n316 = stacked-sequence {
    frame #0 {
      n317 = Wait (ms)(milliseconds to wait=u32 20) -> ()  [unwired: 1 out]
    }
    frame #1 {
      # "调整启动时的前面板尺寸边界"
      # "应当等程序启动之后再执行这一步→_→"
      n318 = Call Chain ("调用链")() -> (call chain=w386:string[])
      n319 = Index Array(array=w386, index=0) -> (element=w384:string)
      n320 = Open VI Reference(vi path=w384) -> (vi reference=w396:refnum<vi>)  [unwired: 1 in, 5 out]
      n321 = property class="VI"(reference=w396) -> ("Front Panel.PanelBounds"=w393:T3)  [unwired: 1 in, 2 out]
      n322 = property class="VI"(reference=w396) -> (reference out=w397:refnum<vi>, "Minimum Panel Size"=w387:T4)  [unwired: 1 in, 1 out]
      n323 = Unbundle By Name(w387) -> ("Horizontal"=w394:i16, "Vertical"=w391:i16)
      n324 = Unbundle By Name(w393) -> ("Left"=w395:i16, "Top"=w390:i16)
      n325 = Add(x=w394, y=w395) -> (x+y=w392:i16)
      n326 = Add(x=w391, y=w390) -> (x+y=w389:i16)
      n327 = Bundle By Name(cluster=w393, "Right"=w392, "Bottom"=w389) -> (w388:T3)
      n328 = property class="VI"(reference=w397, "Front Panel.PanelBounds"=w388) -> (reference out=w398:refnum<vi>)  [unwired: 1 in, 1 out]
      n329 = Close Reference(reference=w398) -> ()  [unwired: 1 in, 1 out]
    }
    frame #2 {
      w401 = i16 0
      # "自动调整窗格原点"
      n330 = property on="Pane" class="Pane"() -> ("Origin"=w400:T4)  [unwired: 2 in, 2 out]
      n331 = Bundle By Name(cluster=w400, "Horizontal"=w401, "Vertical"=w401) -> (w399:T4)
      n332 = property on="Pane" class="Pane"("Origin"=w399) -> ()  [unwired: 2 in, 2 out]
    }
    frame #3 {
      n333 = call "SearchCom.vi"() -> ("下拉列表项"=w402:cluster{"String":string, "Value":i32}[])  [unwired: 3 in]
      n334 = property on="串口号" class="Ring (严格)"("StringsAndValues[]"=w402) -> ()  [unwired: 2 in, 2 out]
      n335 = invoke on="接收文本框:" class="Str" method="Append String"("string"="硬石电子\nhttp://www.ing10bbs.com/\n携手合作,共创未来\n") -> ()  [unwired: 3 in, 4 out]
      n336 = property on="串口号" class="Ring (严格)"("DisabledEnum"=T2."Enabled" ("禁用")) -> ()  [unwired: 2 in, 2 out]
    }
  }
  n337 = while {
    stop <- TRUE continue-if-true
    w406 = u32 300
    n338 = event shown="[1] 菜单选择(用户)" {
      selector: _ -> [_ _]
      dyn-events: _ -> [_ _]
      timeout: w406 -> [_ _]
      event Timeout {
        n339 = event-data() -> ()  [unwired: 1 in, 3 out]
      }
      event Menu Selection (User) {
        n340 = event-data() -> ("ItemTag"=w411:string)  [unwired: 1 in, 1 out]
        n341 = Not Equal?(x="硬石电子出品", y=w411) -> (x != y?=w412:bool)
        n342 = case shown="真" w412 {
          tunnel: w411 -> [_ w414]
          frame False {
          }
          frame True {
            n343 = call-poly <vilib>:"Open URL in Default Browser.vi"("URL"=w414) -> ()  [unwired: 5 in, 2 out]
          }
        }
      }
    }
    n344 = Wait Until Next ms Multiple(millisecond multiple=w406) -> ()  [unwired: 1 out]
    n345 = case shown="真" "刷新按钮" {
      selector: "刷新按钮" -> [_ w409]
      frame False {
      }
      frame True {
        n346 = Not(x=w409) -> (.not. x?=w408:bool)
        n347 = call "SearchCom.vi"("使用注册表？"=w408) -> ("下拉列表项"=w410:cluster{"String":string, "Value":i32}[])  [unwired: 2 in]
        n348 = property on="刷新按钮" class="Bool (严格)"("Value"=w408) -> ()  [unwired: 2 in, 2 out]
        n349 = property on="串口号" class="Ring (严格)"("StringsAndValues[]"=w410) -> ()  [unwired: 2 in, 2 out]
      }
    }
  }
  n350 = property on="串口号" class="Ring (严格)" props=["Value"]() -> ()  [unwired: 2 in, 3 out]
